vi "Items Below Range.vi"(10 "Location Translation":cluster{"dst":i64, "src":i64, "rng":i64}, 11 "Initial Items":cluster{"strt":i64, "rng":i64}) -> (3 "Items Below Range":cluster{"strt":i64, "rng":i64})   [LabVIEW 2023, in "d5.lvlib"]
uses:
  d5.lvlib
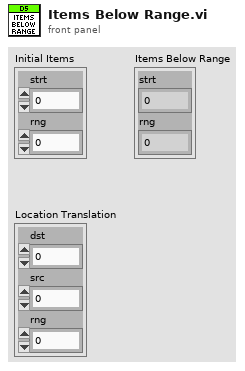
[diagram p1: front panel]
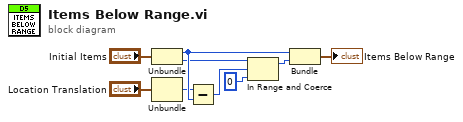
[diagram p0: block diagram]
diagram:
  n1 = Unbundle("Initial Items") -> ("strt"=w7:i64, "rng"=w3:i64)
  n2 = Unbundle("Location Translation") -> ("src"=w6:i64)  [unwired: 2 out]
  n3 = Subtract(x=w6, y=w7) -> (x-y=w4:i64)
  n4 = In Range and Coerce(upper limit=w3, x=w4, lower limit=i64 0 ("x")) -> (coerced(x)=w9:i64)  [unwired: 1 out]
  n5 = Bundle("strt"=w7, "rng"=w9) -> (→"Items Below Range":cluster{"strt":i64, "rng":i64})  [unwired: 1 in]
